vi "NI 9213 TASK.vi"(8 "error in":errorcluster, 11 "MODULE NAME":string="cDAQ_NICOTRAMod4") -> (0 "error out":errorcluster, 3 "task out":refnum<k21>)   [LabVIEW 2016]
uses:
  <vilib>/DAQmx/read.llb/DAQmx Read (Analog 1D DBL NChan 1Samp).vi
  <vilib>/DAQmx/miscellaneous.llb/DAQmx Fill In Error Info.vi
  <vilib>/DAQmx/configure/timing.llb/DAQmx Timing (Sample Clock).vi
  <vilib>/DAQmx/create/channels.llb/DAQmx Create Channel (AI-Temperature-RTD).vi
  <resource>/objmgr/daqmx.rc
  <vilib>/DAQmx/create/channels.llb/DAQmx Create Channel (TEDS-AI-Temperature-Thermocouple).vi
  <vilib>/DAQmx/create/channels.llb/DAQmx Create Channel (AI-Temperature-Thermocouple).vi
panel:
  out "data":dbl[](array[numeric]) format="%0.2f"
  out "Numeric":i32
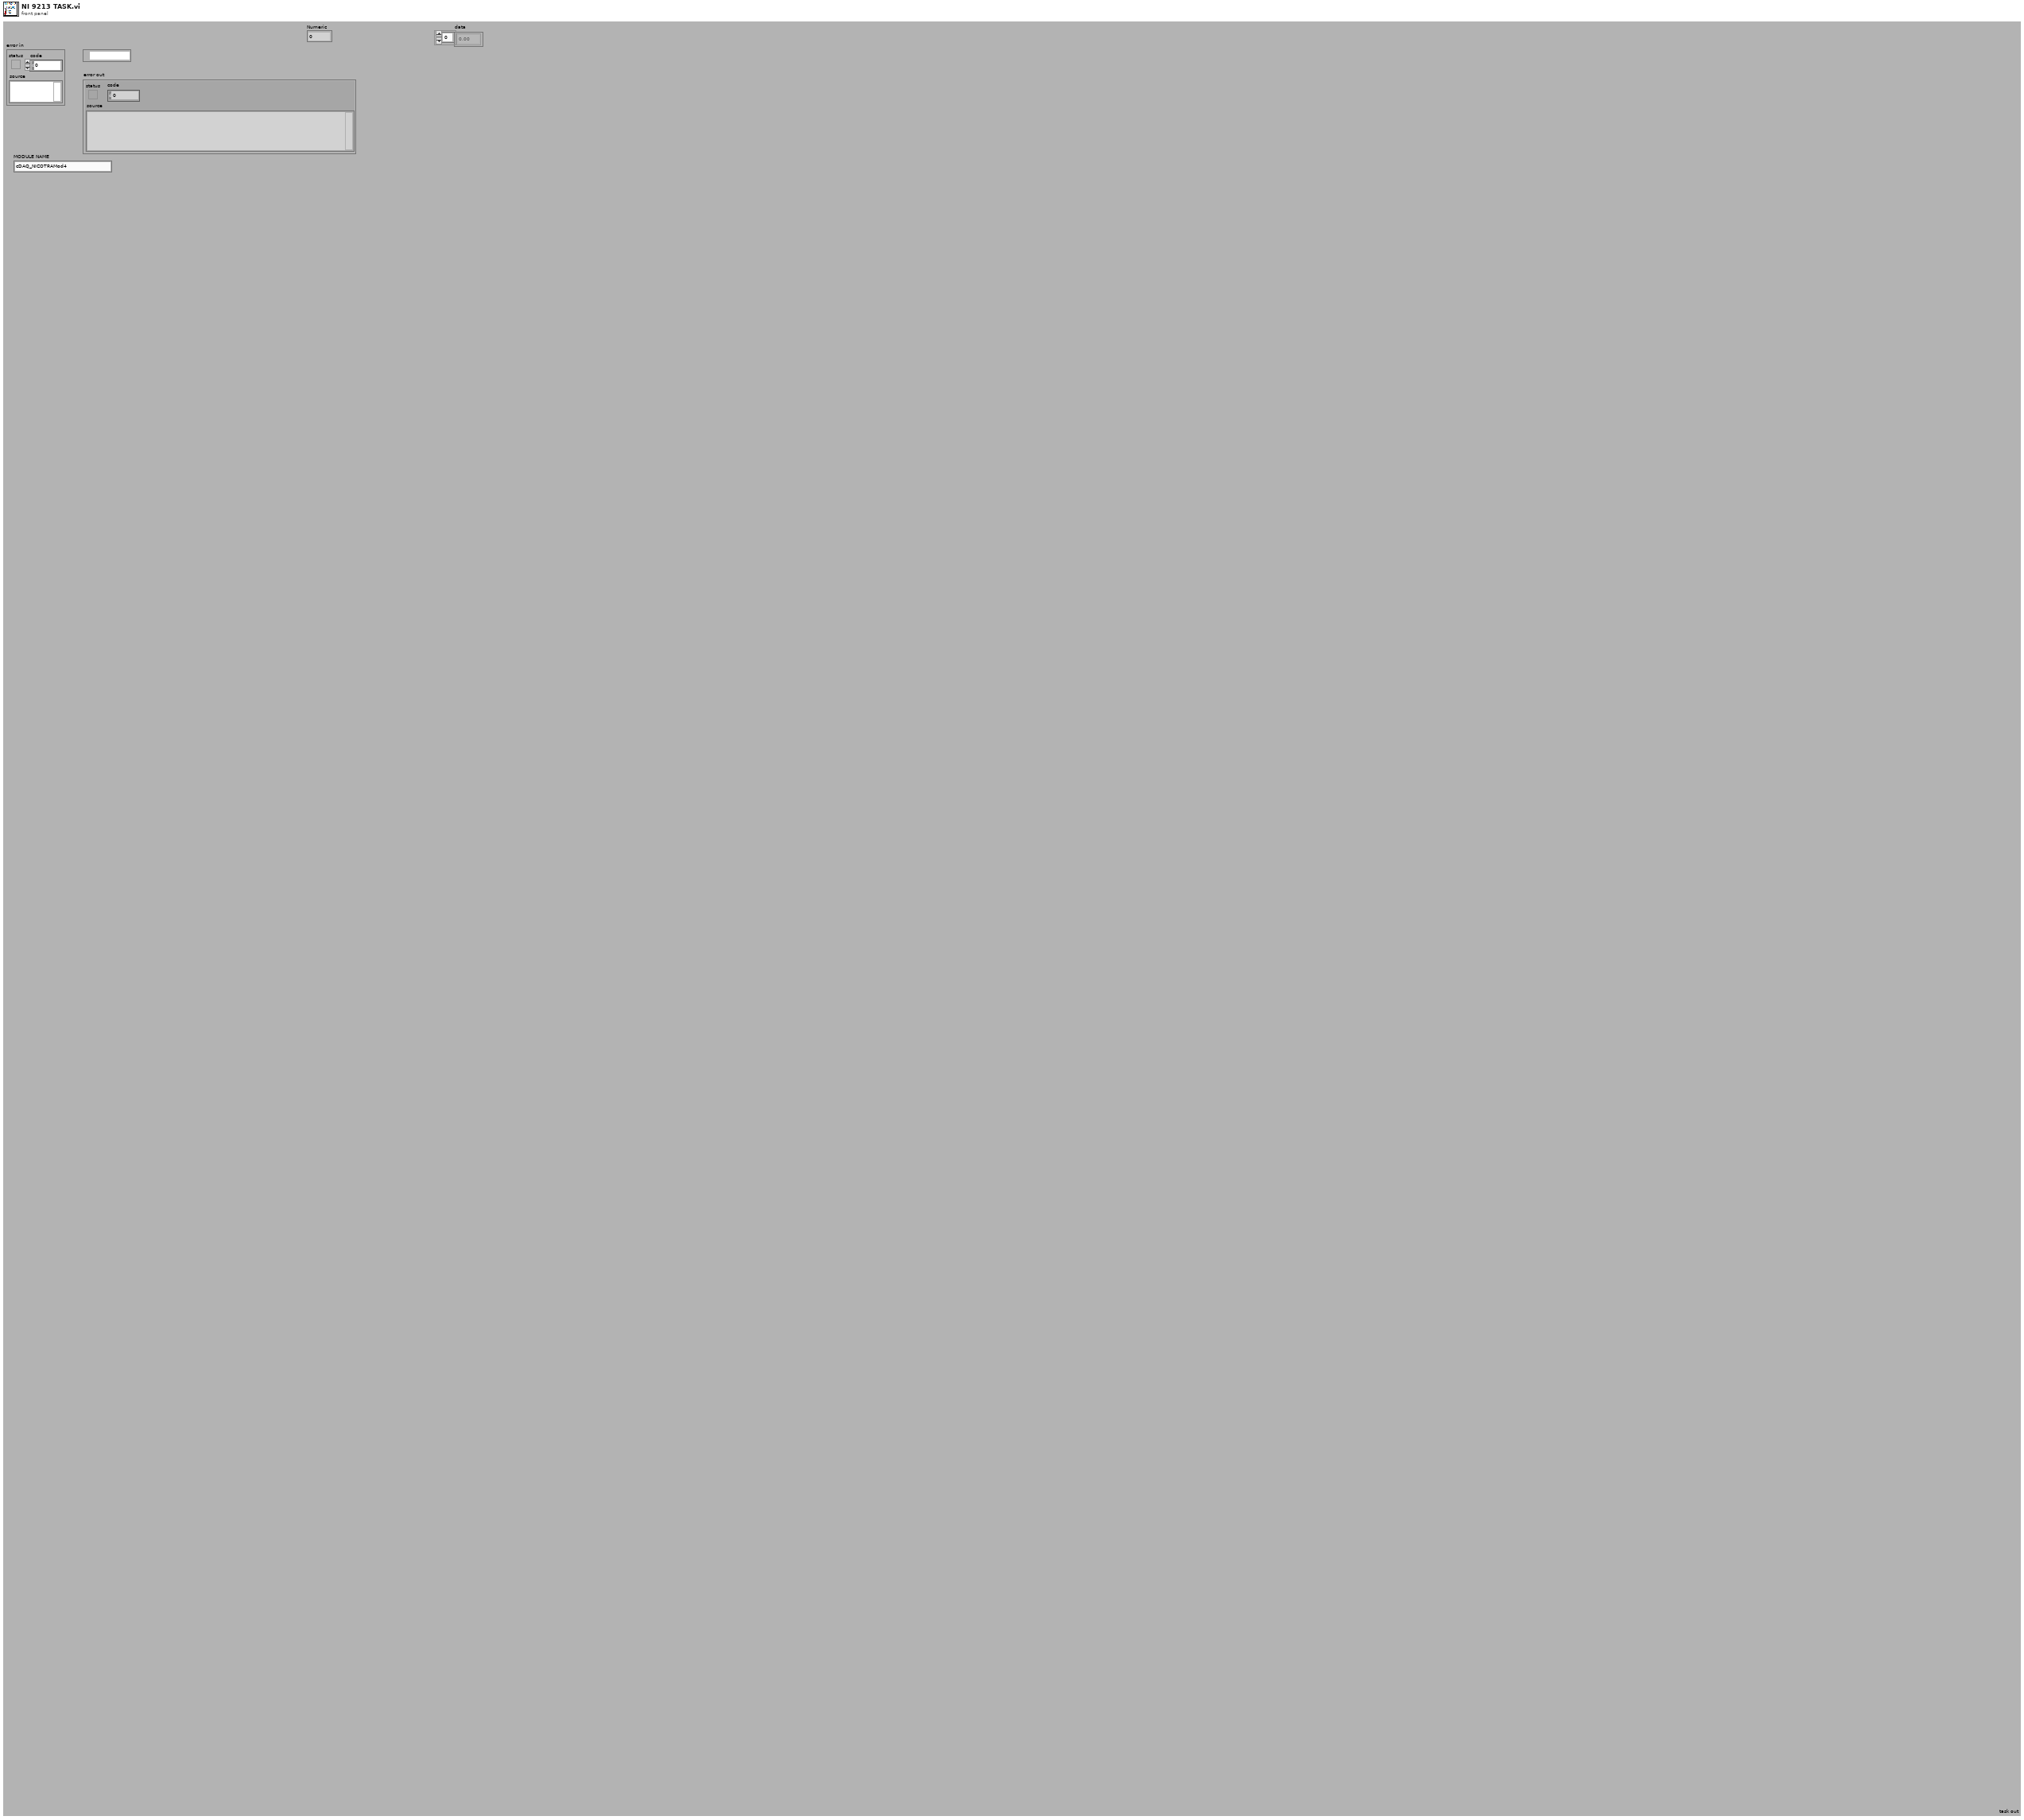
[diagram p1: front panel]
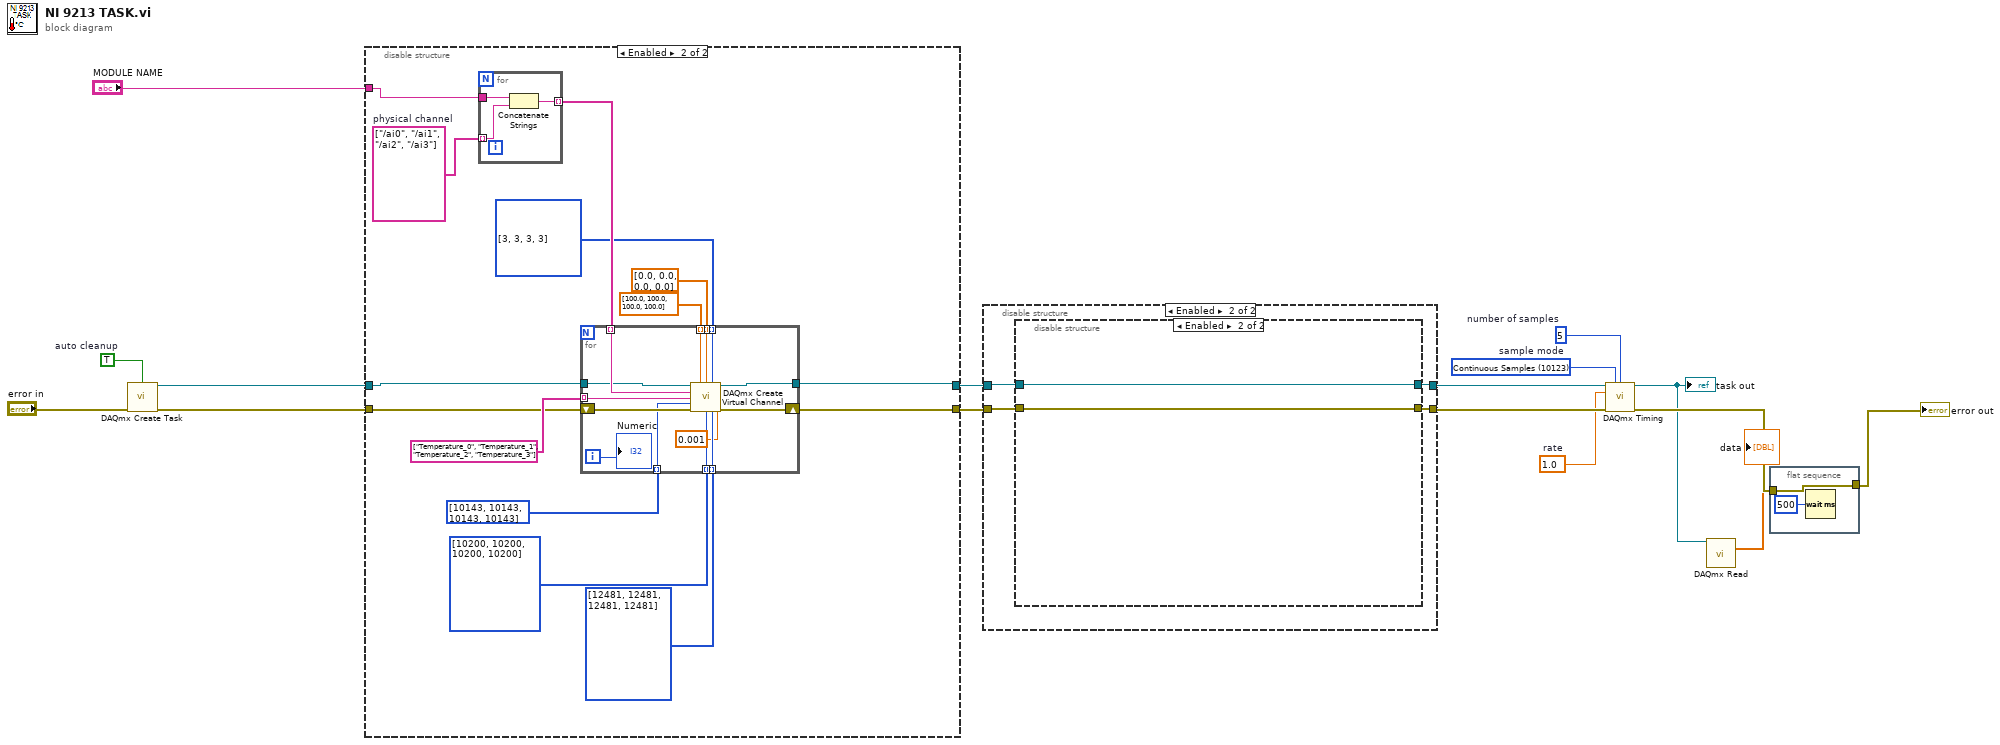
[diagram p0: block diagram]
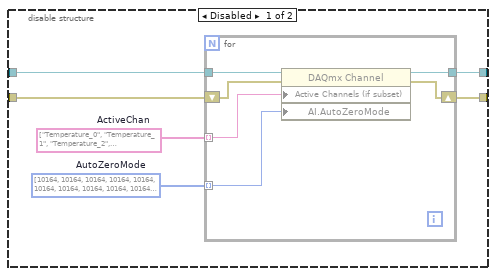
[diagram p2: hidden frame]
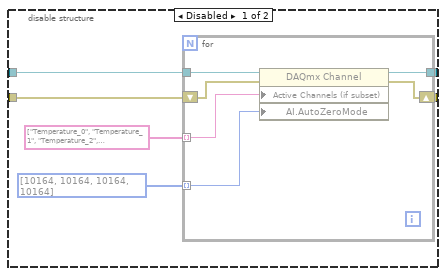
[diagram p3: hidden frame]
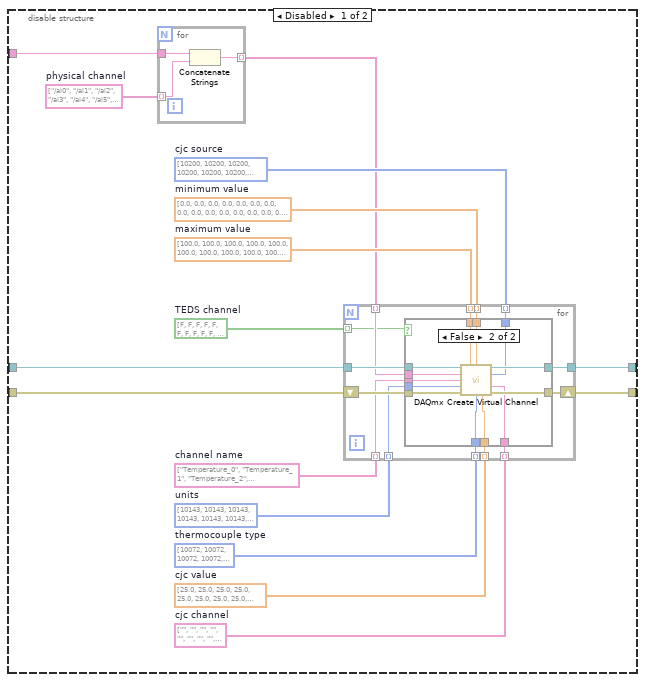
[diagram p4: hidden frame]
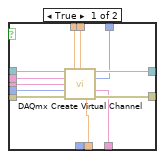
[diagram p5: hidden frame]
diagram:
  w7 = 10123 items=["Finite Samples"=10178, "Continuous Samples"=10123, "Hardware Timed Single Point"=12522]  # sample mode
  w8 = 5  # number of samples
  w9 = 1.0  # rate
  w15 = TRUE  # auto cleanup
  n1 = call <vilib>:"DAQmx Create Task.vi"("auto cleanup"=w15, "error in"="error in") -> ("task out"=w14:refnum<k21>, "error out"=w16:errorcluster)  [unwired: 12 in]
  n2 = disable-structure shown="Enabled" {
    disable-tunnel: w16 -> [w32 w78]
    disable-tunnel: w14 -> [w31 w85]
    disable-tunnel: [w25 w79] -> w13
    disable-tunnel: [w20 w80] -> w11
    disable-tunnel: "MODULE NAME" -> [w18 w87]
    frame Disabled {
      w21 = bool[] [FALSE, FALSE, FALSE, FALSE, FALSE, FALSE, FALSE, FALSE, FALSE, FALSE, FALSE, FALSE, FALSE, FALSE, FALSE, FALSE]  # TEDS channel
      w23 = dbl[] [25.0, 25.0, 25.0, 25.0, 25.0, 25.0, 25.0, 25.0, 25.0, 25.0, 25.0, 25.0, 25.0, 25.0, 25.0, 25.0]  # cjc value
      w22 = string[] ["", "", "", "", "", "", "", "", "", "", "", "", "", "", "", ""]  # cjc channel
      w28 = i32[] [10072, 10072, 10072, 10072, 10072, 10072, 10072, 10072, 10073, 10073, 10073, 10073, 10073, 10073, 10073, 10072] items=["J"=10072, "K"=10073, "N"=10077, "R"=10082, "S"=10085, "T"=10086, "B"=10047, "E"=10055]  # thermocouple type
      w27 = i32[] [10143, 10143, 10143, 10143, 10143, 10143, 10143, 10143, 10143, 10143, 10143, 10143, 10143, 10143, 10143, 10143] items=["deg C"=10143, "deg F"=10144, "Kelvins"=10325, "deg R"=10145, "From Custom Scale"=10065]  # units
      w26 = string[] ["Temperature_0", "Temperature_1", "Temperature_2", "Temperature_3", "Temperature_4", "Temperature_5", "Temperature_6", "Temperature_7", "Temperature_8", "Temperature_9", "Temperature_10", "Temperature_11", "Temperature_12", "Temperature_13", "Temperature_14", "Temperature_15"]  # channel name
      w19 = string[] ["/ai0", "/ai1", "/ai2", "/ai3", "/ai4", "/ai5", "/ai6", "/ai7", "/ai8", "/ai9", "/ai10", "/ai11", "/ai12", "/ai13", "/ai14", "/ai15"]  # physical channel
      w29 = dbl[] [100.0, 100.0, 100.0, 100.0, 100.0, 100.0, 100.0, 100.0, 100.0, 100.0, 100.0, 100.0, 100.0, 100.0, 100.0, 100.0]  # maximum value
      w30 = dbl[] [0.0, 0.0, 0.0, 0.0, 0.0, 0.0, 0.0, 0.0, 0.0, 0.0, 0.0, 0.0, 0.0, 0.0, 0.0, 0.0]  # minimum value
      w24 = u32[] [10200, 10200, 10200, 10200, 10200, 10200, 10200, 10200, 10200, 10200, 10200, 10200, 10200, 10200, 10200, 10200] items=["Internal"=10200, "Constant Value"=10116, "Channel"=10113]  # cjc source
      n3 = for {
        tunnel: w19 -> [w34] mode=indexing
        tunnel: w18 -> [w35]
        tunnel: [w33] -> w17 mode=indexing
        n4 = Concatenate Strings(w35, w34) -> (w33:string)
      }
      n5 = for {
        tunnel: w31 -> [w47]
        tunnel: w30 -> [w48] mode=indexing
        tunnel: w29 -> [w49] mode=indexing
        tunnel: w28 -> [w37] mode=indexing
        tunnel: w27 -> [w41] mode=indexing
        tunnel: w26 -> [w43] mode=indexing
        tunnel: w17 -> [w42] mode=indexing
        tunnel: [w45] -> w20
        tunnel: w24 -> [w40] mode=indexing
        tunnel: w23 -> [w39] mode=indexing
        tunnel: w22 -> [w38] mode=indexing
        shift-right: [w44] -> w25
        shift-left: w32 -> [w46]
        tunnel: w21 -> [w36] mode=indexing
        n6 = case shown="False" w36 {
          tunnel: w49 -> [w61 w74]
          tunnel: w48 -> [w60 w73]
          tunnel: w47 -> [w59 w72]
          tunnel: w46 -> [w58 w71]
          tunnel: [w57 w70] -> w45
          tunnel: [w56 w69] -> w44
          tunnel: w43 -> [w55 w68]
          tunnel: w42 -> [w54 w67]
          tunnel: w41 -> [w53 w66]
          tunnel: w40 -> [w52 w65]
          tunnel: w39 -> [w51 w64]
          tunnel: w38 -> [w50 w63]
          tunnel: w37 -> [_ w62]
          frame True {
            n7 = call-poly <vilib>:"DAQmx Create Virtual Channel.vi"("task in"=w59, "maximum value"=w61, "minimum value"=w60, "physical channels"=w54, "cjc source"=w52, "name to assign"=w55, "units"=w53, "cjc channel"=w50, "error in"=w58, "cjc value"=w51) -> ("task out"=w57:refnum<k21>, "error out"=w56:errorcluster)  [unwired: 4 in]
          }
          frame False {
            n8 = call-poly <vilib>:"DAQmx Create Virtual Channel.vi"("task in"=w72, "maximum value"=w74, "minimum value"=w73, "physical channels"=w67, "cjc source"=w65, "name to assign"=w68, "units"=w66, "cjc channel"=w63, "error in"=w71, "thermocouple type"=w62, "cjc value"=w64) -> ("task out"=w70:refnum<k21>, "error out"=w69:errorcluster)  [unwired: 3 in]
          }
        }
      }
    }
    frame Enabled {
      w76 = i32[] [12481, 12481, 12481, 12481] items=["Pt3750"=12481, "Pt3851"=10071, "Pt3911"=12482, "Pt3916"=10069, "Pt3920"=10053, "Pt3928"=12483, "Custom"=10137]
      w75 = i32[] [10200, 10200, 10200, 10200] items=["Internal"=10200, "External"=10167, "None"=10230]
      w77 = i32[] [10143, 10143, 10143, 10143] items=["Deg C"=10143, "Deg F"=10144, "Kelvins"=10325, "Deg R"=10145, "From Custom Scale"=10065]
      w83 = i32[] [3, 3, 3, 3] items=["2-Wire"=2, "3-Wire"=3, "4-Wire"=4]
      w88 = string[] ["/ai0", "/ai1", "/ai2", "/ai3"]  # physical channel
      n9 = for {
        tunnel: w88 -> [w104] mode=indexing
        tunnel: w87 -> [w105]
        tunnel: [w103] -> w86 mode=indexing
        n10 = Concatenate Strings(w105, w104) -> (w103:string)
      }
      n11 = for {
        tunnel: [w101] -> w80
        shift-right: [w100] -> w79
        shift-left: w78 -> [w102]
        tunnel: w86 -> [w99] mode=indexing
        tunnel: w85 -> [w98]
        tunnel: string[] ["Temperature_0", "Temperature_1", "Temperature_2", "Temperature_3"] -> [w97] mode=indexing
        tunnel: w83 -> [w96] mode=indexing
        tunnel: dbl[] [0.0, 0.0, 0.0, 0.0] -> [w95] mode=indexing
        tunnel: dbl[] [100.0, 100.0, 100.0, 100.0] -> [w94] mode=indexing
        tunnel: w77 -> [w93] mode=indexing
        tunnel: w76 -> [w92] mode=indexing
        tunnel: w75 -> [w91] mode=indexing
        i -> [w90]
        n12 = call-poly <vilib>:"DAQmx Create Virtual Channel.vi"("task in"=w98, "maximum value"=w94, "minimum value"=w95, "resistance configuration"=w96, "physical channels"=w99, "name to assign"=w97, "units"=w93, "current excitation value"=0.001, "error in"=w102, "current excitation source"=w91, "rtd type"=w92) -> ("task out"=w101:refnum<k21>, "error out"=w100:errorcluster)  [unwired: 3 in]
        "Numeric" <- w90
      }
    }
  }
  n13 = disable-structure shown="Enabled" {
    disable-tunnel: w13 -> [w111 w121]
    disable-tunnel: [w109 w118] -> w12
    disable-tunnel: w11 -> [w107 w120]
    disable-tunnel: [w106 w119] -> w10
    frame Disabled {
      w108 = i32[] [10164, 10164, 10164, 10164, 10164, 10164, 10164, 10164, 10164, 10164, 10164, 10164, 10164, 10164, 10164, 10164] items=["None"=10230, "Once"=10244, "Every Sample"=10164]  # AutoZeroMode
      w110 = string[] ["Temperature_0", "Temperature_1", "Temperature_2", "Temperature_3", "Temperature_4", "Temperature_5", "Temperature_6", "Temperature_7", "Temperature_8", "Temperature_9", "Temperature_10", "Temperature_11", "Temperature_12", "Temperature_13", "Temperature_14", "Temperature_15"]  # ActiveChan
      n14 = for {
        tunnel: w107 -> [w115]
        tunnel: w110 -> [w116] mode=indexing
        shift-right: [w117] -> w109
        shift-left: w111 -> [w112]
        tunnel: [w114] -> w106
        tunnel: w108 -> [w113] mode=indexing
        n15 = property class="DAQmx Channel"(reference=w115, error in=w112, "Active Channels (if subset)"=w116, "AI.AutoZeroMode"=w113) -> (reference out=w114:refnum<k21>, error out=w117:errorcluster)
      }
    }
    frame Enabled {
      n16 = disable-structure shown="Enabled" {
        disable-tunnel: w121 -> [w127 w134]
        disable-tunnel: w120 -> [w126 w135]
        disable-tunnel: [w125 w135] -> w119
        disable-tunnel: [w124 w134] -> w118
        frame Disabled {
          w122 = i32[] [10164, 10164, 10164, 10164] items=["None"=10230, "Once"=10244, "Every Sample"=10164]
          n17 = for {
            tunnel: w126 -> [w131]
            tunnel: string[] ["Temperature_0", "Temperature_1", "Temperature_2", "Temperature_3"] -> [w132] mode=indexing
            shift-right: [w133] -> w124
            shift-left: w127 -> [w128]
            tunnel: [w130] -> w125
            tunnel: w122 -> [w129] mode=indexing
            n18 = property class="DAQmx Channel"(reference=w131, error in=w128, "Active Channels (if subset)"=w132, "AI.AutoZeroMode"=w129) -> (reference out=w130:refnum<k21>, error out=w133:errorcluster)
          }
        }
        frame Enabled {
        }
      }
    }
  }
  n19 = call-poly <vilib>:"DAQmx Timing.vi"("task/channels in"=w10, "sample mode"=w7, "samples per channel"=w8, "rate"=w9, "error in"=w12) -> ("task out"=w2:refnum<k21>, "error out"=w4:errorcluster)  [unwired: 9 in]
  "task out" <- w2
  n20 = call-poly <vilib>:"DAQmx Read.vi"("task/channels in"=w2) -> ("data"=→"data":dbl[])  [unwired: 12 in, 2 out]
  n21 = flat-sequence {
    tunnel: [w136] -> w3
    tunnel: w4 -> [w136]
    frame #0 {
      n22 = Wait (ms)(milliseconds to wait=u32 500) -> ()  [unwired: 1 out]
    }
  }
  "error out" <- w3
